vi "ClearColorOf2DListCtrl.vi"(7 "scroll reset?":bool, 9 "Font Color":u32(colorbox)=4018019, 10 "BG Color":u32(colorbox)=4018019, 11 "ArrayRef in":refnum<vi>) -> (3 "ArrayRef out":refnum<vi>)   [LabVIEW 2018, in "Library-Ctrl.lvlib"]
uses:
  Library-Ctrl.lvlib
  <vilib>/Utility/miscctls.llb/LVRowAndColumnUnsignedTypeDef.ctl
  <vilib>/Utility/miscctls.llb/LVRowAndColumnTypeDef.ctl
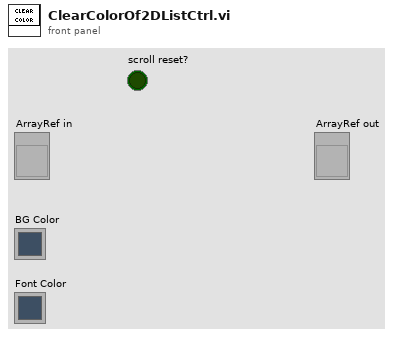
[diagram p1: front panel]
types:
  T1 = typedef "LVRowAndColumnTypeDef.ctl" = cluster{"Row":i32, "Column":i32}
  T2 = typedef "LVRowAndColumnUnsignedTypeDef.ctl" = cluster{"Row":u32, "Column":u32}
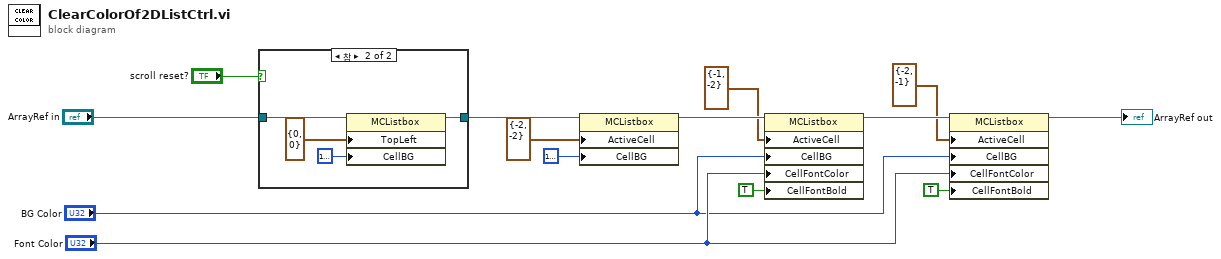
[diagram p0: block diagram]
diagram:
  n1 = case shown="참" "scroll reset?" {
    tunnel: "ArrayRef in" -> [w15 w18]
    tunnel: [w15 w17] -> w13
    frame False {
    }
    frame True {
      n2 = property class="MCListbox"(reference=w18, "TopLeft"=T2 {"Row"=0, "Column"=0} ("왼쪽 위에 보이는 셀"), "CellBG"=u32 16777226 ("Font Color")) -> (reference out=w17:refnum<vi>)  [unwired: 1 in, 1 out]
    }
  }
  n3 = property class="MCListbox"(reference=w13, "ActiveCell"=T1 {"Row"=-2, "Column"=-2} ("활성 셀:활성 셀"), "CellBG"=u32 16777226 ("Font Color")) -> (reference out=w11:refnum<vi>)  [unwired: 1 in, 1 out]
  n4 = property class="MCListbox"(reference=w11, "ActiveCell"=T1 {"Row"=-1, "Column"=-2} ("활성 셀:활성 셀"), "CellBG"="BG Color", "CellFontColor"="Font Color", "CellFontBold"=TRUE ("활성 셀:셀 폰트:굵은체")) -> (reference out=w9:refnum<vi>)  [unwired: 1 in, 1 out]
  n5 = property class="MCListbox"(reference=w9, "ActiveCell"=T1 {"Row"=-2, "Column"=-1} ("활성 셀:활성 셀"), "CellBG"="BG Color", "CellFontColor"="Font Color", "CellFontBold"=TRUE ("활성 셀:셀 폰트:굵은체")) -> (reference out=→"ArrayRef out":refnum<vi>)  [unwired: 1 in, 1 out]
